vi "Agilent B2900 Series Output Sweep Volts.vi"() -> ()   [LabVIEW 2023]
doc: "This example shows how to use the instrument's output voltage sweep mode. The actual voltage levels and actual current levels are returned as well as whether over current protection (OCP) has been tripped."
uses:
  Agilent B2900 Series.lvlib
  Public/Data/Low Level/Fetch Measurement (Multiple Points).vi
  Public/Configure/Measurement/Configure Measurement (Current).vi
panel:
  in  "Compliance Current (0.0001 A)":dbl=0.0001
  in  "Sweep Number of Steps (1)":i32=1
  in  "Sweep Range Mode (2: Auto)":i32(ring)=2 items=["Best", "Fix", "Auto"]
  in  "Sweep Stop (10 V)":dbl=10.0
  in  "Sweep Start (3 V)":dbl=3.0
  in  "Sweep Output Mode (0: Linear Single)":i32(ring) items=["Linear Single", "Linear Double", "Log Single", "Log Double"]
  out "Actual Voltage Levels (V)":dbl[](array[numeric])
  out "Actual Current Levels (A)":dbl[](array[numeric])
  out "OCP Tripped?":bool
  in  "Current NPLC (0.1)":dbl=0.1
  in  "Trigger Source (0: Auto-Internal)":i32(ring) items=["Auto-Internal", "Bus", "Timer", "INT1", "INT2", "LAN", "EXT1", "EXT2", "EXT3", "EXT4", "EXT5", "EXT6", "EXT7", "EXT8", "EXT9", "EXT10", "EXT11", "EXT12", "EXT13", "EXT14"]
  in  "Enable Output Protection(T: Enable)":bool=TRUE
  in  "Channel (0: Channel 1)":i32(ring) items=["Channel 1", "Channel 2"]
  in  "VISA resource name":refnum<visa-resource-name>
  # "(c) 2011-2021 National Instruments.  ALL RIGHTS RESERVED."
  # "Output Settings"
  # "Compliance Protection"
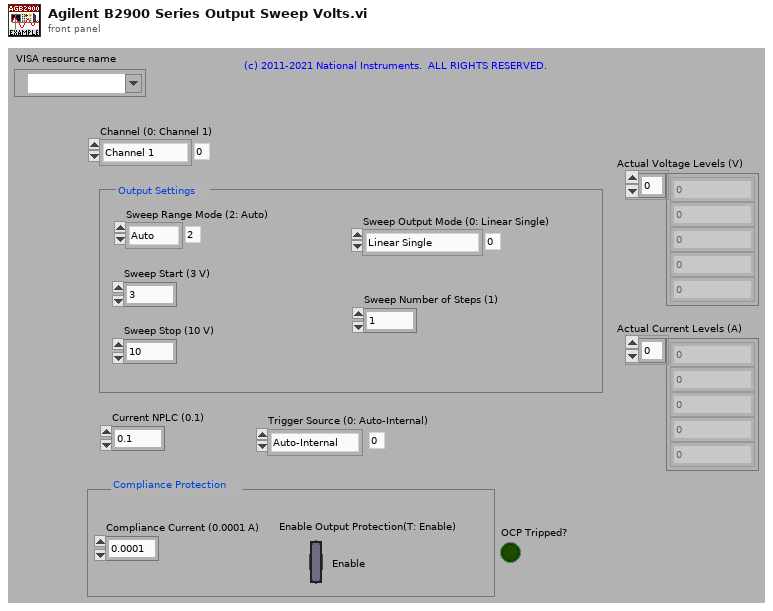
[diagram p1: front panel]
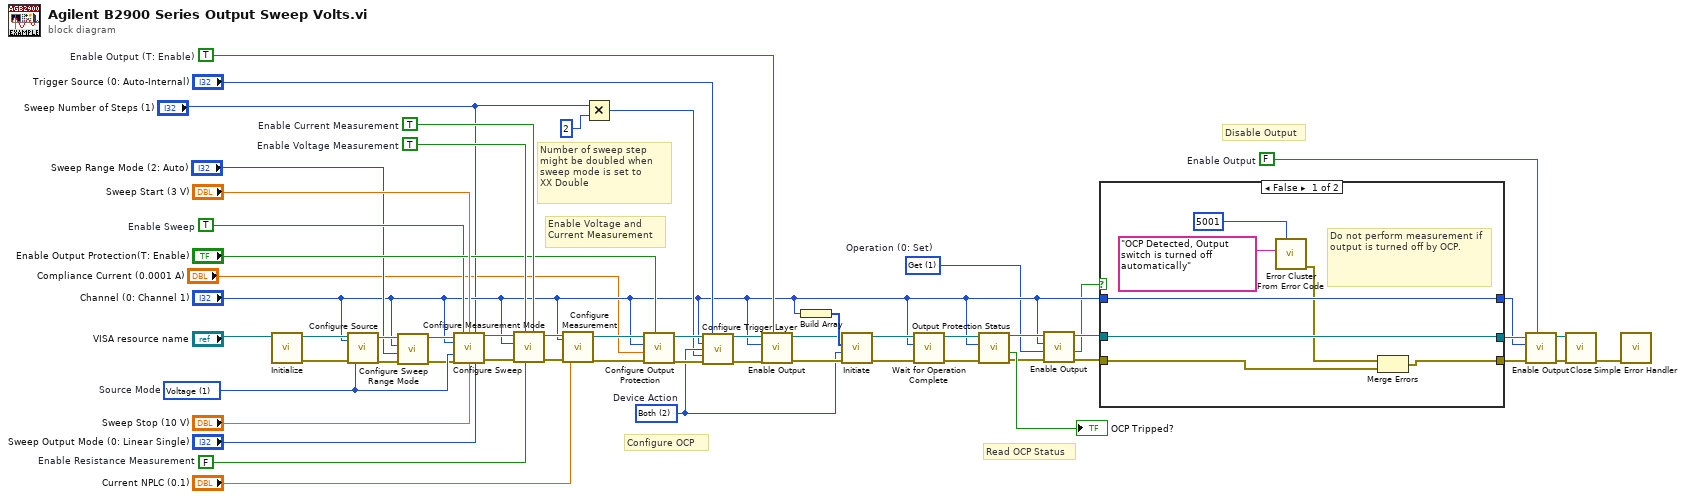
[diagram p0: block diagram]
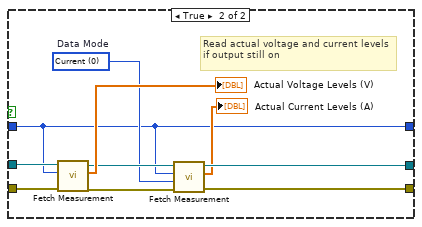
[diagram p2: hidden frame]
diagram:
  w5 = 1 items=["Set", "Get"]  # Operation (0: Set)
  w27 = TRUE  # Enable Current Measurement
  w28 = TRUE  # Enable Voltage Measurement
  w50 = FALSE  # Enable Output
  w26 = 2 items=["Acquire", "Transient", "Both"]  # Device Action
  w31 = FALSE  # Enable Resistance Measurement
  w22 = 1 items=["Current", "Voltage"]  # Source Mode
  w18 = TRUE  # Enable Sweep
  w55 = TRUE  # Enable Output (T: Enable)
  # "Number of sweep step \nmight be doubled when \nsweep mode is set to \nXX Double"
  # "Disable Output"
  # "Read OCP Status"
  # "Enable Voltage and \nCurrent Measurement"
  # "Configure OCP"
  n1 = call "Initialize.vi"("VISA resource name"="VISA resource name") -> ("error out"=w29:errorcluster, "VISA resource name out"=w30:refnum<visa-resource-name>)  [unwired: 9 in]
  n2 = call "Configure Source.vi"("VISA resource name"=w30, "Channel (0: Channel 1)"="Channel (0: Channel 1)", "error in (no error)"=w29, "Source Mode (1: Voltage)"=w22) -> ("VISA resource name out"=w17:refnum<visa-resource-name>, "error out"=w14:errorcluster)  [unwired: 14 in]
  n3 = call "Configure Sweep Range Mode.vi"("error in (no error)"=w14, "Sweep Range Mode (2: Auto)"="Sweep Range Mode (2: Auto)", "Channel (0: Channel 1)"="Channel (0: Channel 1)", "VISA resource name"=w17) -> ("error out"=w15:errorcluster, "VISA resource name out"=w16:refnum<visa-resource-name>)  [unwired: 6 in]
  n4 = call "Configure Sweep.vi"("VISA resource name"=w16, "Enable Sweep (F: Disable)"=w18, "Sweep Start (0)"="Sweep Start (3 V)", "Sweep Number of Steps (1)"="Sweep Number of Steps (1)", "Channel (0: Channel 1)"="Channel (0: Channel 1)", "Sweep Setting Mode (1: Voltage)"=w22, "error in (no error)"=w15, "Sweep Stop (0)"="Sweep Stop (10 V)", "Sweep Output Mode (0: Linear Single)"="Sweep Output Mode (0: Linear Single)") -> ("VISA resource name out"=w20:refnum<visa-resource-name>, "error out"=w19:errorcluster)  [unwired: 5 in]
  n5 = call "Configure Measurement Mode.vi"("Enable Current Measurement (T: Enable)"=w27, "Enable Resistance Measurement (F: Disable)"=w31, "Enable Voltage Measurement (T: Enable)"=w28, "error in (no error)"=w19, "Channel (0: Channel 1)"="Channel (0: Channel 1)", "VISA resource name"=w20) -> ("error out"=w51:errorcluster, "VISA resource name out"=w52:refnum<visa-resource-name>)  [unwired: 4 in]
  n6 = call-poly "Configure Measurement.vi"("VISA resource name"=w52, "Channel (0: Channel 1)"="Channel (0: Channel 1)", "error in (no error)"=w51, "Current NPLC (0.1)"="Current NPLC (0.1)") -> ("VISA resource name out"=w39:refnum<visa-resource-name>, "error out"=w38:errorcluster)  [unwired: 14 in]
  n7 = Multiply(x="Sweep Number of Steps (1)", y=2) -> (x*y=w24:i32)
  n8 = call "Configure Output Protection.vi"("Enable Output Protection (T: Enable)"="Enable Output Protection(T: Enable)", "error in (no error)"=w38, "Compliance Current (0.0001 A)"="Compliance Current (0.0001 A)", "Channel (0: Channel 1)"="Channel (0: Channel 1)", "VISA resource name"=w39) -> ("error out"=w36:errorcluster, "VISA resource name out"=w37:refnum<visa-resource-name>)  [unwired: 5 in]
  n9 = call "Configure Trigger Layer.vi"("VISA resource name"=w37, "Trigger Source (0: Auto-Internal)"="Trigger Source (0: Auto-Internal)", "Channel (0: Channel 1)"="Channel (0: Channel 1)", "Device Action (2: Both)"=w26, "Trigger Count (1)"=w24, "error in (no error)"=w36) -> ("VISA resource name out"=w35:refnum<visa-resource-name>, "error out"=w34:errorcluster)  [unwired: 8 in]
  n10 = call "Enable Output.vi"("Enable Output (F: Disable)"=w55, "error in (no error)"=w34, "Channel (0: Channel 1)"="Channel (0: Channel 1)", "VISA resource name"=w35) -> ("error out"=w53:errorcluster, "VISA resource name out"=w54:refnum<visa-resource-name>)  [unwired: 5 in, 1 out]
  n11 = Build Array("Channel (0: Channel 1)") -> (w56:i32[])
  n12 = call "Initiate.vi"("error in (no error)"=w53, "Device Action (2: Both)"=w26, "Channel List ({Channel1})"=w56, "VISA resource name"=w54) -> ("error out"=w32:errorcluster, "VISA resource name out"=w33:refnum<visa-resource-name>)  [unwired: 6 in]
  n13 = call "Wait for Operation Complete.vi"("error in (no error)"=w32, "Channel (0: Channel 1)"="Channel (0: Channel 1)", "VISA resource name"=w33) -> ("error out"=w42:errorcluster, "VISA resource name out"=w43:refnum<visa-resource-name>)  [unwired: 7 in]
  n14 = call "Output Protection Status.vi"("error in (no error)"=w42, "Channel (0: Channel 1)"="Channel (0: Channel 1)", "VISA resource name"=w43) -> ("error out"=w7:errorcluster, "OCP Tripped?"=→"OCP Tripped?":bool, "VISA resource name out"=w10:refnum<visa-resource-name>)  [unwired: 5 in, 1 out]
  n15 = call "Enable Output.vi"("error in (no error)"=w7, "Operation (0: Set)"=w5, "Channel (0: Channel 1)"="Channel (0: Channel 1)", "VISA resource name"=w10) -> ("error out"=w9:errorcluster, "Output Enabled?"=w4:bool, "VISA resource name out"=w8:refnum<visa-resource-name>)  [unwired: 5 in]
  n16 = case shown="False" w4 {
    tunnel: w8 -> [w63 w73]
    tunnel: w9 -> [w58 w72]
    tunnel: [w60 w71] -> w41
    tunnel: [w63 w68] -> w40
    tunnel: "Channel (0: Channel 1)" -> [w64 w65]
    tunnel: [w64 w65] -> w12
    frame False {
      # "Do not perform measurement if output is turned off by OCP."
      n17 = call <vilib>:"Error Cluster From Error Code.vi"("error message (\"\")"="OCP Detected, Output switch is turned off automatically" ("error message (\"\")"), "error code (0)"=5001) -> ("error out"=w59:errorcluster)  [unwired: 7 in]
      n18 = Merge Errors(w59, w58) -> (w60:errorcluster)
    }
    frame True {
      w67 = 0 items=["Current", "Resistance", "Source Output Setting", "Status", "Time", "Voltage"]  # Data Mode
      # "Read actual voltage and current levels if output still on"
      n19 = call-poly "Fetch Measurement.vi"("error in (no error)"=w72, "Channel (0: Channel 1)"=w65, "VISA resource name"=w73) -> ("error out"=w70:errorcluster, "Measurements"=→"Actual Voltage Levels (V)":dbl[], "VISA resource name out"=w69:refnum<visa-resource-name>)  [unwired: 6 in]
      n20 = call-poly "Fetch Measurement.vi"("error in (no error)"=w70, "Data Mode (5: Voltage)"=w67, "Channel (0: Channel 1)"=w65, "VISA resource name"=w69) -> ("error out"=w71:errorcluster, "Measurements"=→"Actual Current Levels (A)":dbl[], "VISA resource name out"=w68:refnum<visa-resource-name>)  [unwired: 5 in]
    }
  }
  n21 = call "Enable Output.vi"("Enable Output (F: Disable)"=w50, "error in (no error)"=w41, "Channel (0: Channel 1)"=w12, "VISA resource name"=w40) -> ("error out"=w46:errorcluster, "VISA resource name out"=w45:refnum<visa-resource-name>)  [unwired: 5 in, 1 out]
  n22 = call "Close.vi"("error in (no error)"=w46, "VISA resource name"=w45) -> ("error out"=w47:errorcluster)  [unwired: 9 in]
  n23 = call <vilib>:"Simple Error Handler.vi"("error in (no error)"=w47) -> ()  [unwired: 4 in, 5 out]
